vi "LS4 Disconnect_SD.vi"() -> (0 "Command executed":bool)   [LabVIEW 2015]
doc: "This VI must be used to close the connection to the LStep control. It closes the interface and deallocates memory."
uses:
  DLL/LStep4.dll
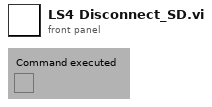
[diagram p1: front panel]
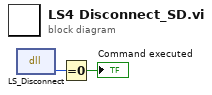
[diagram p0: block diagram]
diagram:
  n1 = dll-call lib="G:/SD/TRANCON-2015/DLL/LStep4.dll" fn="LS_Disconnect"() -> ("type de retour"=w2:i32)  [unwired: 3 in, 2 out]
  n2 = Equal To 0?(x=w2) -> (x = 0?=→"Command executed":bool)
